vi "Clear OLED.vi"(8 "error in (no error)":errorcluster, 11 "64x128 I2C OLED SSD1315 in":refnum<class "48x64 I2C OLED SSD1306.lvclass">) -> (0 "error out":errorcluster, 2 "2D Picture":picture, 3 "64x128 I2C OLED SSD1315 out":refnum<class "48x64 I2C OLED SSD1306.lvclass">)   [LabVIEW 2020, in "CTI-Peripheral.lvlib" / "48x64 I2C OLED SSD1306.lvclass"]
uses:
  48x64 I2C OLED SSD1306.lvclass
  48x64 I2C OLED SSD1306.lvclass/48x64 I2C OLED SSD1306.ctl
  CTI/I2C Connection/I2C Connection.lvclass/I2C Connection.ctl
  GetPicture.vi
  BuildMessagesFromPicture.vi
  CTI/Session/I2C Write Data.vi
  CTI/I2C Connection/I2C Connection.lvclass
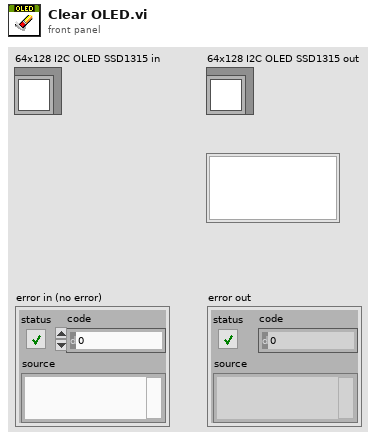
[diagram p1: front panel]
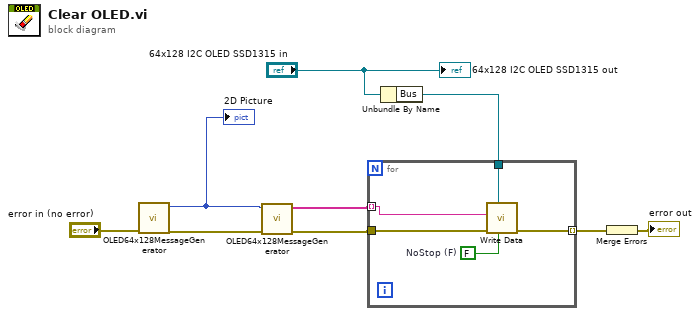
[diagram p0: block diagram]
diagram:
  n1 = call-poly "OLED64x128MessageGenerator.vi"("error in (no error)"="error in (no error)") -> ("error out"=w5:errorcluster, "2D Picture"=w4:picture)  [unwired: 9 in]
  "2D Picture" <- w4
  n2 = call-poly "OLED64x128MessageGenerator.vi"("error in (no error)"=w5, "2D Picture"=w4) -> ("error out"=w2:errorcluster, "Messages"=w3:string[])  [unwired: 8 in]
  n3 = Unbundle By Name("64x128 I2C OLED SSD1315 in") -> ("Bus"=w7:refnum<class "I2C Connection.lvclass">)
  n4 = for {
    tunnel: w7 -> [w13]
    tunnel: w3 -> [w10] mode=indexing
    tunnel: w2 -> [w11]
    tunnel: [w14] -> w9 mode=indexing
    w12 = FALSE  # NoStop (F)
    n5 = call "Write Data.vi"("NoStop (F)"=w12, "I2C Connection"=w13, "error in (no error)"=w11, "Data"=w10) -> ("error out"=w14:errorcluster)  [unwired: 7 in]
  }
  n6 = Merge Errors(w9) -> (→"error out":errorcluster)
  "64x128 I2C OLED SSD1315 out" <- "64x128 I2C OLED SSD1315 in"
